vi "Set Temperature.vi"(8 "error in (no error)":errorcluster, 10 "Temperature setpoint":dbl min=0.0 max=1000.0 format="%#.1f", 11 "Temperature Controller in":refnum<class "Mercury Temperature Controller.lvclass">) -> (0 "error out":errorcluster, 3 "Temperature Controller out":refnum<class "Mercury Temperature Controller.lvclass">)   [LabVIEW 2015, in "Mercury Temperature Controller.lvclass"]
uses:
  Mercury Temperature Controller.lvclass
  maglab ultrasound -- arkady/mercury ixx/public/Controls/Unit String.ctl
  maglab ultrasound -- arkady/mercury ixx/public/Controls/Comms Transport Layer.ctl
  maglab ultrasound -- arkady/mercury ixx/public/Controls/ISOBus Address.ctl
  Mercury Temperature Controller.lvclass/Mercury Temperature Controller.ctl
  maglab ultrasound -- arkady/mercury ixx/public/libraries/Temperature/Open/Open Temperature Device.vi
  maglab ultrasound -- arkady/mercury ixx/public/libraries/Temperature/Configuration/Read/Temperature Device (Read).vi
  maglab ultrasound -- arkady/mercury ixx/public/libraries/control loop/configuration/Set/Temperature Setpoint (Set).vi
  maglab ultrasound -- arkady/mercury ixx/Mercury iXX.lvlib
  maglab ultrasound -- arkady/mercury ixx/public/libraries/Temperature.lvlib
  maglab ultrasound -- arkady/mercury ixx/public/libraries/Control Loop.lvlib
  maglab ultrasound -- arkady/mercury ixx/public/libraries/System.lvlib
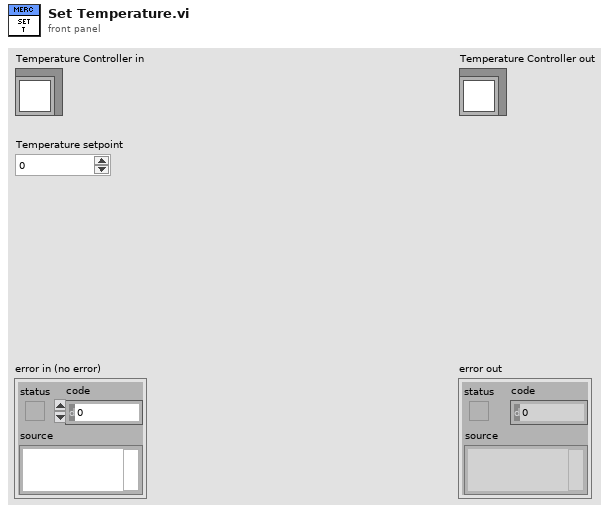
[diagram p1: front panel]
types:
  T1 = typedef "Mercury iXX.lvlib/Comms Transport Layer.ctl" = enum16{"Ethernet TCP/IP", "USB", "ISOBus - RS-232", "GPIB"}
  T2 = typedef "Mercury iXX.lvlib/Unit String.ctl" = string
  T3 = typedef "Mercury iXX.lvlib/ISOBus Address.ctl" = i32
  T4 = typedef "Mercury iXX.lvlib/Mercury Reference.ctl" = cluster{"Comms":refnum<visa-resource-name>, "Device ID":string[], "Comms Layer":T1, "Command":string, "Query reference":T5}
  T5 = typedef "Mercury iXX.lvlib/Query Dynamic Reference.ctl" = refnum<vi>
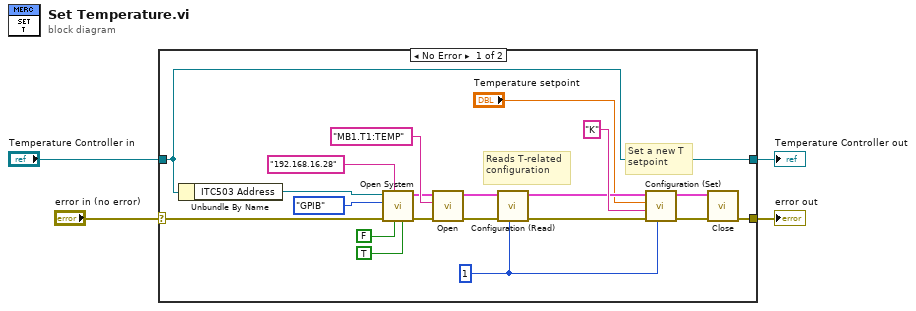
[diagram p0: block diagram]
diagram:
  n1 = case shown="No Error" "error in (no error)" {
    selector: "error in (no error)" -> [w5 w26]
    tunnel: [w7 w26] -> w3
    tunnel: [w18 w25] -> w1
    tunnel: "Temperature Controller in" -> [w18 w25]
    frame No Error {
      w10 = T3 1 ("ISOBUS address")
      # "Set a new T setpoint"
      # "Reads T-related configuration"
      n2 = Unbundle By Name(w18) -> ("ITC503 Address"=w12:refnum<visa-resource-name>)
      n3 = call "Open System.vi"("Clear Previous Connections (False)"=TRUE, "ID Query (True)"=FALSE, "IP Address"="192.168.16.28", "error in (no error)"=w5, "Comms Layer"=Comms_Transport_Layer."GPIB", "VISA resource name"=w12) -> ("error out"=w11:errorcluster, "Mercury Reference Out"=w13:T4)  [unwired: 1 in, 3 out]
      n4 = call-poly "Open.vi"("error in (no error)"=w11, "Device Identifier"="MB1.T1:TEMP", "Mercury Reference In"=w13) -> ("error out"=w21:errorcluster, "Mercury Reference Out"=w22:T4)  [unwired: 7 out]
      n5 = call-poly "Configuration (Read).vi"("ISOBUS address"=w10, "error in"=w21, "Mercury Reference In"=w22) -> ("error out"=w20:errorcluster, "Mercury Reference Out"=w19:T4)  [unwired: 7 out]
      n6 = call-poly "Configuration (Set).vi"("ISOBUS address"=w10, "error in"=w20, "Unit"=T2 "K", "Temperature setpoint"="Temperature setpoint", "Mercury Reference In"=w19) -> ("error out"=w8:errorcluster, "Mercury Reference Out"=w6:T4)  [unwired: 3 in, 2 out]
      n7 = call "Close.vi"("error in (no error)"=w8, "Mercury Reference"=w6) -> ("error out"=w7:errorcluster)  [unwired: 9 out]
    }
    frame Error {
    }
  }
  "error out" <- w3
  "Temperature Controller out" <- w1
